vi "CAM_ID_FileSave.vi"(8 "error in":errorcluster, 11 "CAM_ID":T1) -> ()   [LabVIEW 2020]
uses:
  CAM_ID.ctl
  <vilib>/Utility/xml.llb/Write to XML File(string).vi
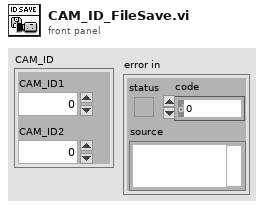
[diagram p1: front panel]
types:
  T1 = typedef "CAM_ID.ctl" = cluster{"CAM_ID1":i32, "CAM_ID2":i32}
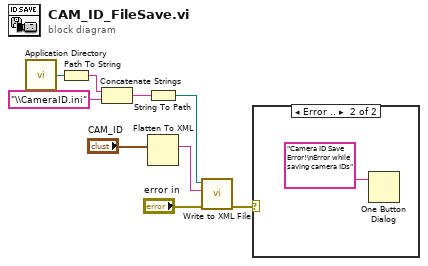
[diagram p0: block diagram]
diagram:
  n1 = call <vilib>:"Application Directory.vi"() -> ("Application Directory"=w7:path)
  n2 = Path To String(path=w7) -> (string=w8:string)
  n3 = Concatenate Strings(w8, "\\CameraID.ini" ("string")) -> (w5:string)
  n4 = String To Path(string=w5) -> (path=w4:path)
  n5 = Flatten To XML(6:"CAM_ID") -> (2:w9:string)
  n6 = call-poly <vilib>:"Write to XML File.vi"("error in (no error)"="error in", "XML Input"=w9, "XML File Path"=w4) -> ("error out"=w1:errorcluster)  [unwired: 6 in, 2 out]
  n7 = case shown="Error .." w1 {
    frame No Error {
    }
    frame Error {
      n8 = One Button Dialog(message="Camera ID Save Error!\nError while saving camera IDs") -> ()  [unwired: 1 in, 1 out]
    }
  }
